vi "Write Verify and Check-in Msg.vi"(10 "Guest Manager UI.lvlib:Verify and Check-in Msg.lvclass":refnum<class "Verify and Check-in Msg.lvclass">, 11 "Guest Manager UI in":refnum<class "Guest Manager UI.lvclass">) -> (3 "Guest Manager UI out":refnum<class "Guest Manager UI.lvclass">)   [LabVIEW 2023, in "Guest Manager UI.lvlib" / "Guest Manager UI.lvclass"]
uses:
  Guest Manager UI.lvclass
  Guest Manager UI Messages/Verify and Check-in Msg/Verify and Check-in Msg.lvclass
  Guest Manager UI.lvclass/Guest Manager UI.ctl
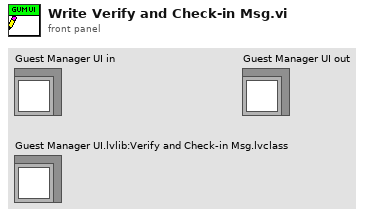
[diagram p1: front panel]
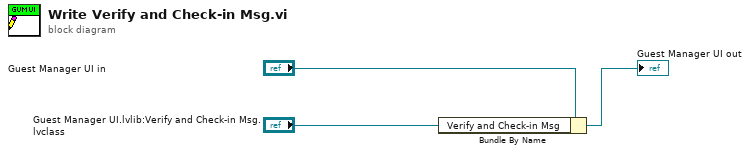
[diagram p0: block diagram]
diagram:
  n1 = Bundle By Name(cluster="Guest Manager UI in", "Verify and Check-in Msg"="Guest Manager UI.lvlib:Verify and Check-in Msg.lvclass") -> (→"Guest Manager UI out":refnum<class "Guest Manager UI.lvclass">)
